vi "Log in.vi"(8 "error in":errorcluster, 11 "log":string) -> (0 "error out":errorcluster)   [LabVIEW 2023]
doc: "Programm läuft string gemacht und alles\nMario Bosnjak\n01.10.2025"
panel:
  out "time string":string
  out "date string":string
  out "Application Directory":path
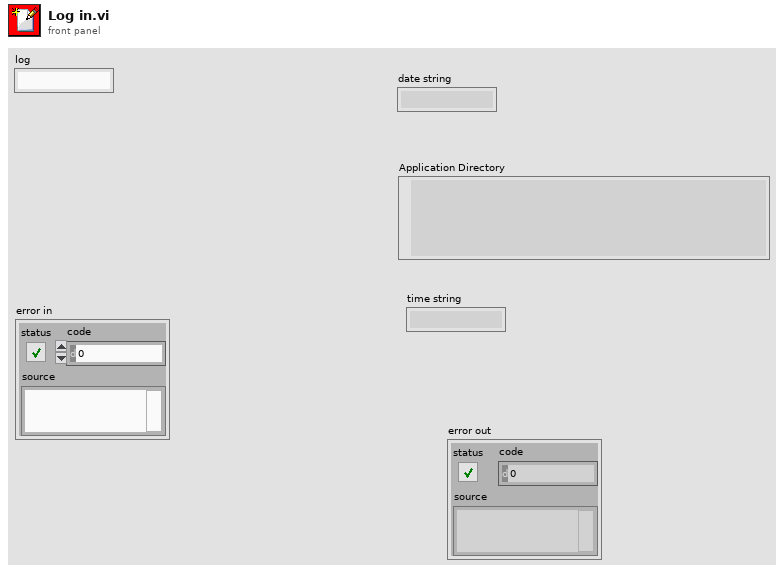
[diagram p1: front panel]
types:
  T1 = enum16{"open", "replace", "create", "open or create", "replace or create", "replace or create with confirmation"}
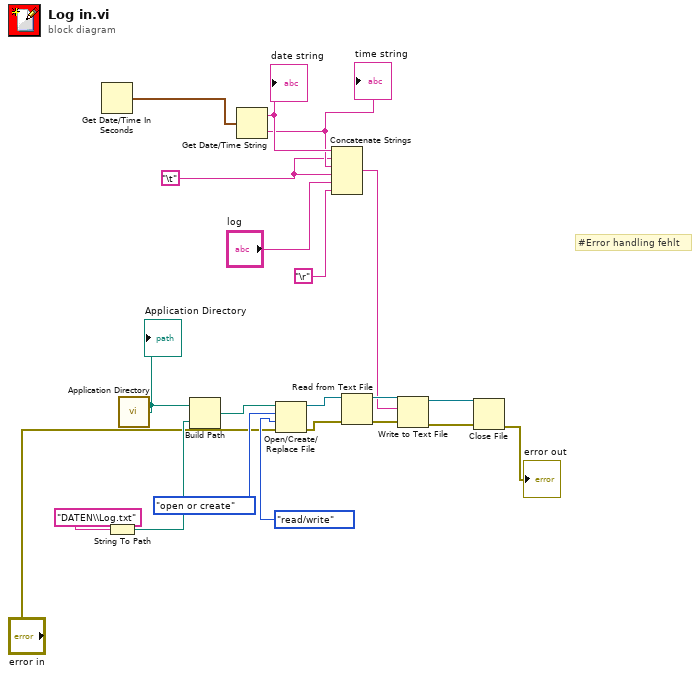
[diagram p0: block diagram]
diagram:
  w5 = "\t"
  # "#Error handling fehlt"
  n1 = Get Date/Time In Seconds() -> (seconds since 1Jan1904=w8:timestamp)
  n2 = String To Path(string="DATEN\\Log.txt") -> (path=w20:path)
  n3 = call <vilib>:"Application Directory.vi"() -> ("Application Directory"=w16:path)
  "Application Directory" <- w16
  n4 = Build Path(base path=w16, name or relative path=w20) -> (appended path=w21:path)
  n5 = Get Date/Time String(seconds (now)=w8) -> (date string=w7:string, time string=w6:string)  [unwired: 2 in]
  "date string" <- w7
  "time string" <- w6
  n6 = Open/Create/Replace File(file path (use dialog)=w21, error in="error in", operation (0:open)=T1."open or create", access (0:read/write)=enum16{"read/write", "read-only", "write-only"}."read/write") -> (refnum out=w13:refnum<file>, error out=w12:errorcluster)  [unwired: 2 in, 1 out]
  n7 = Concatenate Strings(w7, w5, w6, w5, "log", "\r") -> (w9:string)
  n8 = Read from Text File(file (use dialog)=w13, error in=w12) -> (refnum out=w14:refnum<file>, error out=w15:errorcluster)  [unwired: 2 in, 2 out]
  n9 = Write to Text File(file (use dialog)=w14, text=w9, error in=w15) -> (refnum out=w11:refnum<file>, error out=w10:errorcluster)  [unwired: 1 in, 1 out]
  n10 = Close File(refnum=w11, error in=w10) -> (error out=→"error out":errorcluster)  [unwired: 1 out]
